vi "SftpEnumeratePrograms.vi"(0 "error in":errorcluster, 11 "Sftp":refnum<k24>) -> (4 "error out":errorcluster, 15 "Programs":string[](array[string]))   [LabVIEW 2015, in "UnderAutomation.UniversalRobots.lvlib"]
uses:
  UnderAutomation.UniversalRobots.lvlib
  C:/Users/fg/Documents/UniversalRobots.vi/LabVIEW_2024/UnderAutomation.UniversalRobots/lib/UnderAutomation.UniversalRobots.dll
  LabVIEW_2024/UnderAutomation.UniversalRobots/lib/UnderAutomation.UniversalRobots.dll
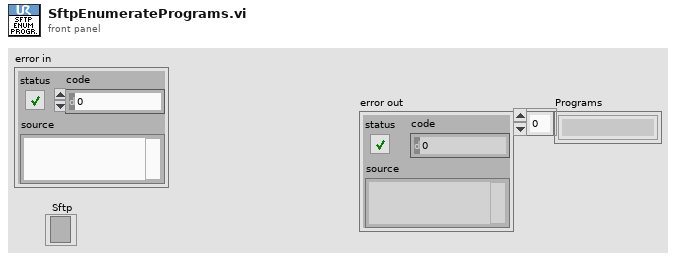
[diagram p1: front panel]
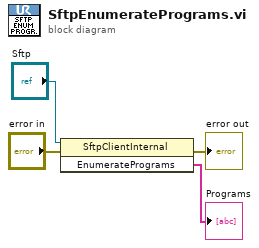
[diagram p0: block diagram]
diagram:
  n1 = invoke class="SftpClientInternal" method="EnumeratePrograms"(reference="Sftp", error in="error in") -> (error out=→"error out":errorcluster, "EnumeratePrograms"=→"Programs":string[])  [unwired: 1 in, 1 out]
